vi "HttpNet_error.vi"(5 "ShowCallChain [T]":bool=TRUE, 6 "IncludedString":string, 7 "OverrideExistingErrors [T]":bool=TRUE, 8 "Error In":errorcluster, 11 "Error":T1) -> (0 "Error Out":errorcluster)   [LabVIEW 2018, in "HttpClient_NET.lvlib"]
doc: "<b> </b> <b> </b>\nHttpClient_NET\nJustin Young - Viviota\nCopyright (c) 2021\nLicense: BSD"
uses:
  HttpClient_NET.lvlib
  Types/HttpNet_error_enum.ctl
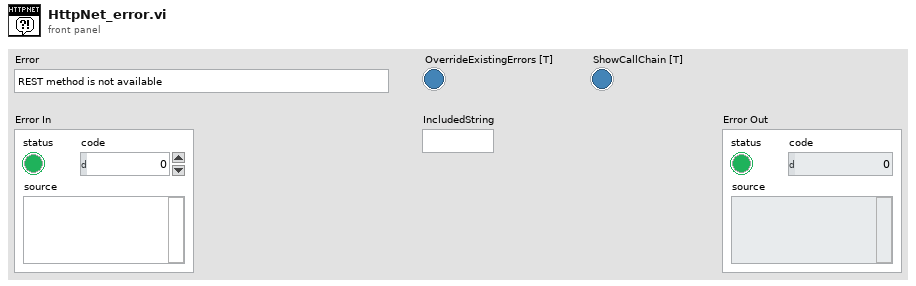
[diagram p1: front panel]
types:
  T1 = typedef "HttpClient_NET.lvlib/HttpNet_error_enum.ctl" = enum16{"REST method is not available", "URL cannot be blank", "Output filepath cannot be empty", "Input filepath cannot be empty", "Internal .NET error %s", "Output filepath cannot be directory", "Download Task no longer exists", "Mutipart Put not supported from REST Client Interface.  Please revert to lower level classes"}
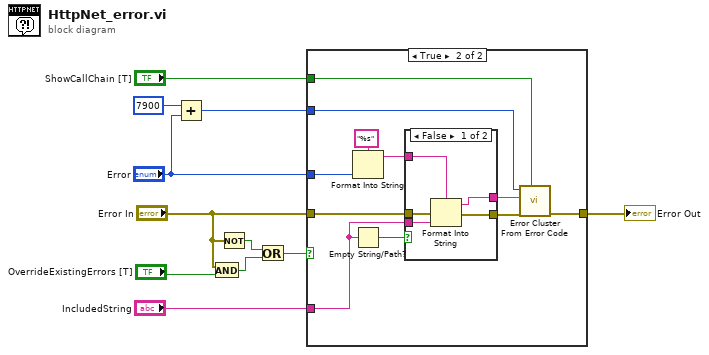
[diagram p0: block diagram]
diagram:
  n1 = Add(x=7900, y="Error") -> (x+y=w10:i32)
  n2 = And(x="Error In", y="OverrideExistingErrors [T]") -> (x .and. y?=w3:bool)
  n3 = Not(x="Error In") -> (.not. x?=w4:bool)
  n4 = Or(x=w4, y=w3) -> (x .or. y?=w2:bool)
  n5 = case shown="True" w2 {
    tunnel: w10 -> [_ w21]
    tunnel: "Error" -> [_ w23]
    tunnel: "Error In" -> [w12 w18]
    tunnel: "ShowCallChain [T]" -> [_ w20]
    tunnel: [w12 w19] -> w7
    tunnel: "IncludedString" -> [_ w13]
    frame False {
    }
    frame True {
      n6 = Format Into String(format string="%s", w23) -> (resulting string=w16:string)  [unwired: 2 in, 1 out]
      n7 = Empty String/Path?(string/path=w13) -> (empty?=w14:bool)
      n8 = case shown="False" w14 {
        tunnel: w18 -> [w28 w29]
        tunnel: [w27 w29] -> w17
        tunnel: w16 -> [w26 w30]
        tunnel: [w25 w30] -> w15
        tunnel: w13 -> [w24 _]
        frame False {
          n9 = Format Into String(format string=w26, error in=w28, w24) -> (resulting string=w25:string, error out=w27:errorcluster)  [unwired: 1 in]
        }
        frame True {
        }
      }
      n10 = call <vilib>:"Error Cluster From Error Code.vi"("show call chain? (False)"=w20, "error in (no error)"=w17, "error message (\"\")"=w15, "error code (0)"=w21) -> ("error out"=w19:errorcluster)  [unwired: 5 in]
    }
  }
  "Error Out" <- w7
